vi "caseStructureExample.vi"() -> ()   [LabVIEW 2014]
panel:
  in  "String Selector":i32
  in  "Input String":string
  out "Result":string
  in  "Boolean Control\n(Modify String If True)":bool
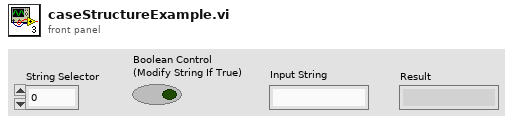
[diagram p1: front panel]
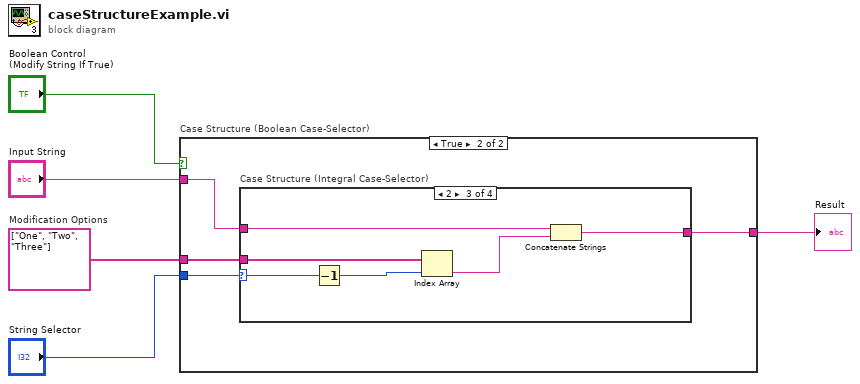
[diagram p0: block diagram]
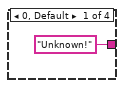
[diagram p3: hidden frame]
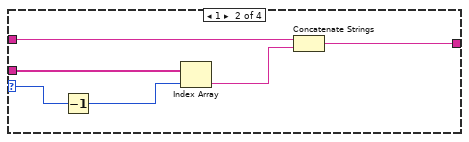
[diagram p4: hidden frame]
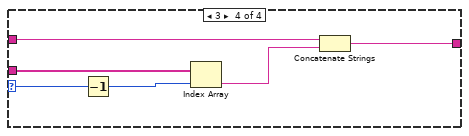
[diagram p5: hidden frame]
diagram:
  w2 = string[] ["One", "Two", "Three"]  # Modification Options
  n1 = case "Case Structure (Boolean Case-Selector)" shown="True" "Boolean Control\n(Modify String If True)" {
    tunnel: [w6 w10] -> w4
    tunnel: "Input String" -> [w6 w7]
    tunnel: w2 -> [_ w9]
    tunnel: "String Selector" -> [_ w8]
    frame False {
    }
    frame True {
      n2 = case "Case Structure (Integral Case-Selector)" shown="2" w8 {
        selector: w8 -> [_ w16 w22 w28]
        tunnel: w9 -> [_ w17 w23 w29]
        tunnel: ["Unknown!" w12 w18 w24] -> w10
        tunnel: w7 -> [_ w14 w20 w26]
        frame 0, Default {
        }
        frame 1 {
          n3 = Decrement(x=w16) -> (x-1=w15:i32)
          n4 = Index Array "Index Array"(array=w17, index=w15) -> (element=w13:string)
          n5 = Concatenate Strings "Concatenate Strings"(w14, w13) -> (w12:string)
        }
        frame 2 {
          n6 = Decrement(x=w22) -> (x-1=w21:i32)
          n7 = Index Array(array=w23, index=w21) -> (element=w19:string)
          n8 = Concatenate Strings(w20, w19) -> (w18:string)
        }
        frame 3 {
          n9 = Decrement(x=w28) -> (x-1=w27:i32)
          n10 = Index Array(array=w29, index=w27) -> (element=w25:string)
          n11 = Concatenate Strings(w26, w25) -> (w24:string)
        }
      }
    }
  }
  "Result" <- w4
